vi "Get Query (as Variant Attributes).vi"(8 "error in (no error)":errorcluster, 10 "Container (default: new variant)":variant, 11 "URI in":refnum<class "URI.lvclass">) -> (0 "error out":errorcluster, 2 "Container with Query Attributes":variant, 3 "URI out":refnum<class "URI.lvclass">)   [LabVIEW 2013, in "openURI.lvlib" / "URI.lvclass"]
doc: "The Query variant input must contain attributes of type \"string\".\nAll data contained in the variant will be ignored. All attributes that are not of type \"string\" will be ignored."
uses:
  URI.lvclass
  URI.lvclass/URI.ctl
  components/query/URI-Component.Query.lvclass/URI-Component.Query.ctl
  components/query/URI-Component.Query.lvclass
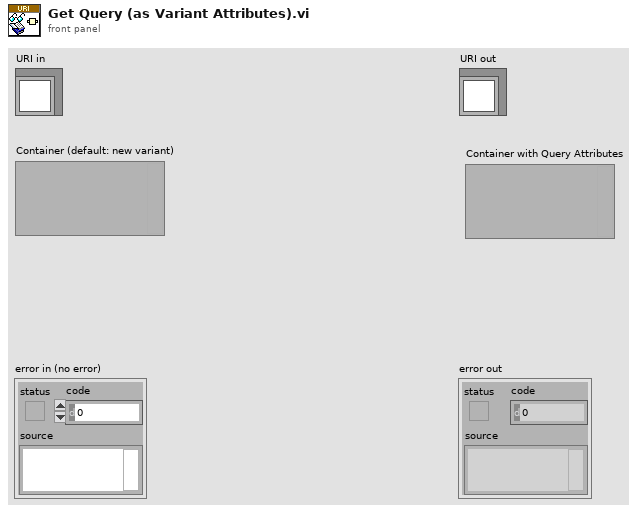
[diagram p1: front panel]
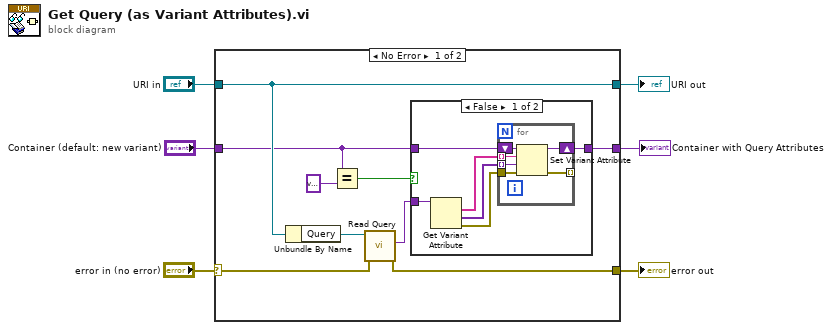
[diagram p0: block diagram]
diagram:
  n1 = case shown="No Error" "error in (no error)" {
    selector: "error in (no error)" -> [w13 w31]
    tunnel: [w12 w31] -> w5
    tunnel: [w15 w30] -> w3
    tunnel: "URI in" -> [w15 w30]
    tunnel: [w7 w29] -> w2
    tunnel: "Container (default: new variant)" -> [w9 w29]
    frame No Error {
      n2 = Unbundle By Name(w15) -> ("Query"=w14:refnum<class "URI-Component.Query.lvclass">)
      n3 = Equal?(x=w9, y=variant) -> (x = y?=w10:bool)
      n4 = call "Read Query.vi"("error in (no error)"=w13, "URI-Component.Query in"=w14) -> ("error out"=w12:errorcluster, "Query"=w8:variant)  [unwired: 7 in, 1 out]
      n5 = case shown="False" w10 {
        tunnel: w9 -> [w20 _]
        tunnel: w8 -> [w21 w28]
        tunnel: [w19 w28] -> w7
        frame False {
          n6 = Get Variant Attribute(Variant=w21) -> (names=w18:string[], values=w17:variant[], error out=w16:errorcluster)  [unwired: 3 in, 1 out]
          n7 = for {
            shift-right: [w26] -> w19
            shift-left: w20 -> [w27]
            tunnel: w18 -> [w25] mode=indexing
            tunnel: w17 -> [w24] mode=indexing
            tunnel: w16 -> [w23]
            tunnel: [w22] -> _ mode=indexing
            n8 = Set Variant Attribute(Variant=w27, name=w25, value=w24, error in=w23) -> (Variant out=w26:variant, error out=w22:errorcluster)  [unwired: 1 out]
          }
        }
        frame True {
        }
      }
    }
    frame Error {
    }
  }
  "error out" <- w5
  "URI out" <- w3
  "Container with Query Attributes" <- w2
